vi "MergeZs.vi"() -> ()   [LabVIEW 2022 SP3]
uses:
  <vilib>/Utility/file.llb/Read From Spreadsheet File (DBL).vi
  <vilib>/Utility/file.llb/Write To Spreadsheet File (DBL).vi
panel:
  in  "Save Data":bool
  out "output array":dbl[][](array[numeric])
  in  "Ring":u16(ring)
  out "subarray 2":dbl[](array[numeric])
  out "subarray":dbl[](array[numeric])
  out "XY Graph":cluster{dbl[], dbl[]}[](graph)
  in  "Use Selected Files":bool
  in  "Listbox":i32[](listbox)
  in  "Choose Directory":path
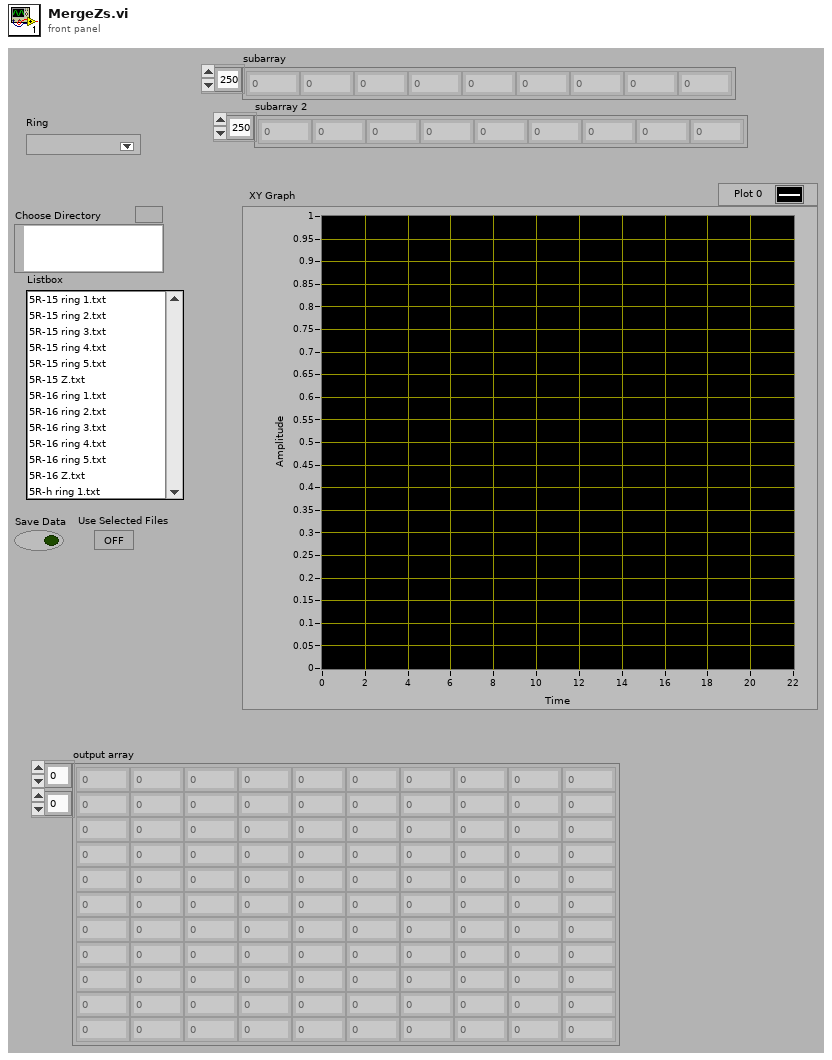
[diagram p1: front panel]
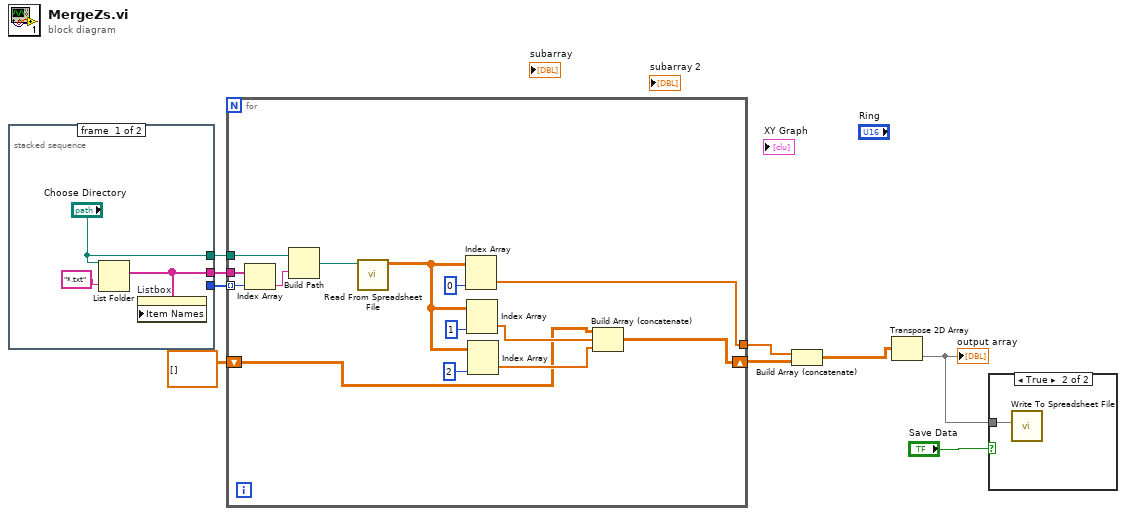
[diagram p0: block diagram]
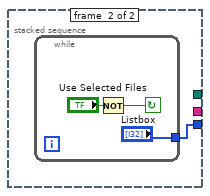
[diagram p3: hidden frame]
diagram:
  n1 = stacked-sequence {
    tunnel: [w11 _] -> w9
    tunnel: [_ w13] -> w8
    tunnel: ["Choose Directory" _] -> w7
    frame #0 {
      n2 = List Folder(path="Choose Directory", pattern="*.txt") -> (filenames=w11:string[])  [unwired: 1 in, 4 out]
      n3 = property on="Listbox" class="LstBox (strict)"("Item Names"=w11) -> ()  [unwired: 2 in, 2 out]
    }
    frame #1 {
      n4 = while {
        tunnel: ["Listbox"] -> w13
        stop <- w15 continue-if-true
        n5 = Not(x="Use Selected Files") -> (.not. x?=w15:bool)
      }
    }
  }
  n6 = for {
    tunnel: w9 -> [w30]
    tunnel: w8 -> [w29] mode=indexing
    tunnel: w7 -> [w27]
    shift-right: [w19] -> w3
    shift-left: dbl[][] [] -> [w18]
    tunnel: [w17] -> w2
    n7 = Index Array(array=w30, index=w29) -> (element=w28:string)
    n8 = Build Path(base path=w27, name or relative path=w28) -> (appended path=w26:path)
    n9 = call-poly <vilib>:"Read From Spreadsheet File.vi"("file path (dialog if empty)"=w26) -> ("all rows"=w22:dbl[][])  [unwired: 6 in, 4 out]
    n10 = Index Array(array=w22, index (col)=0 ("disabled index (col)")) -> (element=w17:dbl[])  [unwired: 1 in]
    n11 = Index Array(array=w22, index (col)=1 ("disabled index (col)")) -> (element=w20:dbl[])  [unwired: 1 in]
    n12 = Index Array(array=w22, index (col)=2 ("disabled index (col)")) -> (element=w21:dbl[])  [unwired: 1 in]
    n13 = Build Array (concatenate)(w18, w20, w21) -> (w19:dbl[][])
  }
  n14 = Build Array (concatenate)(w2, w3) -> (w1:dbl[][])
  n15 = Transpose 2D Array(2D array=w1) -> (transposed array=w6:dbl[][])
  "output array" <- w6
  n16 = case shown="True" "Save Data" {
    tunnel: w6 -> [_ w31]
    frame False {
    }
    frame True {
      n17 = call-poly <vilib>:"Write To Spreadsheet File.vi"("2D data"=w31) -> ()  [unwired: 5 in, 3 out]
    }
  }
